vi "Probe.vi"(8 "error in (no error)":errorcluster, 10 "Buffer":u8[](array[numeric]), 11 "string in":refnum<class "string.lvclass">) -> (0 "error out":errorcluster, 1 "Valid":bool, 2 "Buffer Count":i32, 3 "string out":refnum<class "string.lvclass">)   [LabVIEW 2020, in "Protobuf RAW.lvlib" / "string.lvclass"]
uses:
  string.lvclass
  string.lvclass/string.ctl
  Read String.vi
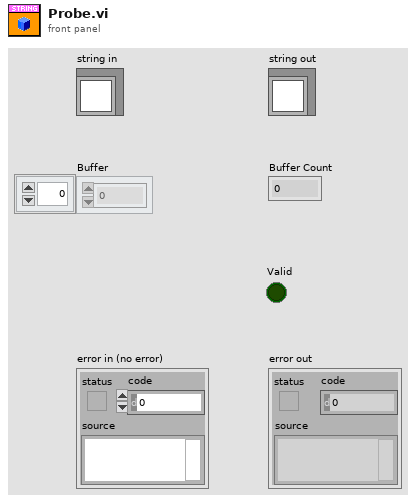
[diagram p1: front panel]
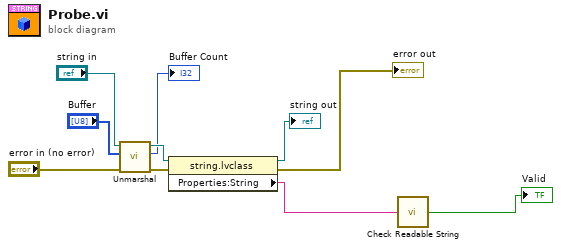
[diagram p0: block diagram]
diagram:
  n1 = call-dynamic "Unmarshal.vi"("error in (no error)"="error in (no error)", "Buffer"="Buffer", "int32 in"="string in") -> ("error out"=w6:errorcluster, "Buffer Count"=→"Buffer Count":i32, "int32 out"=w9:refnum<class "string.lvclass">)  [unwired: 6 in]
  n2 = property class="string.lvclass"(reference=w9, error in=w6) -> (reference out=→"string out":refnum<class "string.lvclass">, error out=→"error out":errorcluster, "Properties:String"=w3:string)
  n3 = call "Check Readable String.vi"("String"=w3) -> ("Valid"=→"Valid":bool)
